vi "HTML_Build_Header_Include_Filelist.vi"(7 "rel. links (f) / include source in .html (T)":bool, 8 "Error In":errorcluster, 10 "abs Path to files on disk":path) -> (0 "Error Out":errorcluster, 1 "<head> JS":string, 2 "<head> CSS":string, 4 "JS_Scripts-Elements":string[](array[string]), 6 "CSS_Links-Elements":string[](array[string]))   [LabVIEW 2014]
uses:
  controls/HTML_Tag_Type.ctl
  controls/StylingFrameworks_Enum.ctl
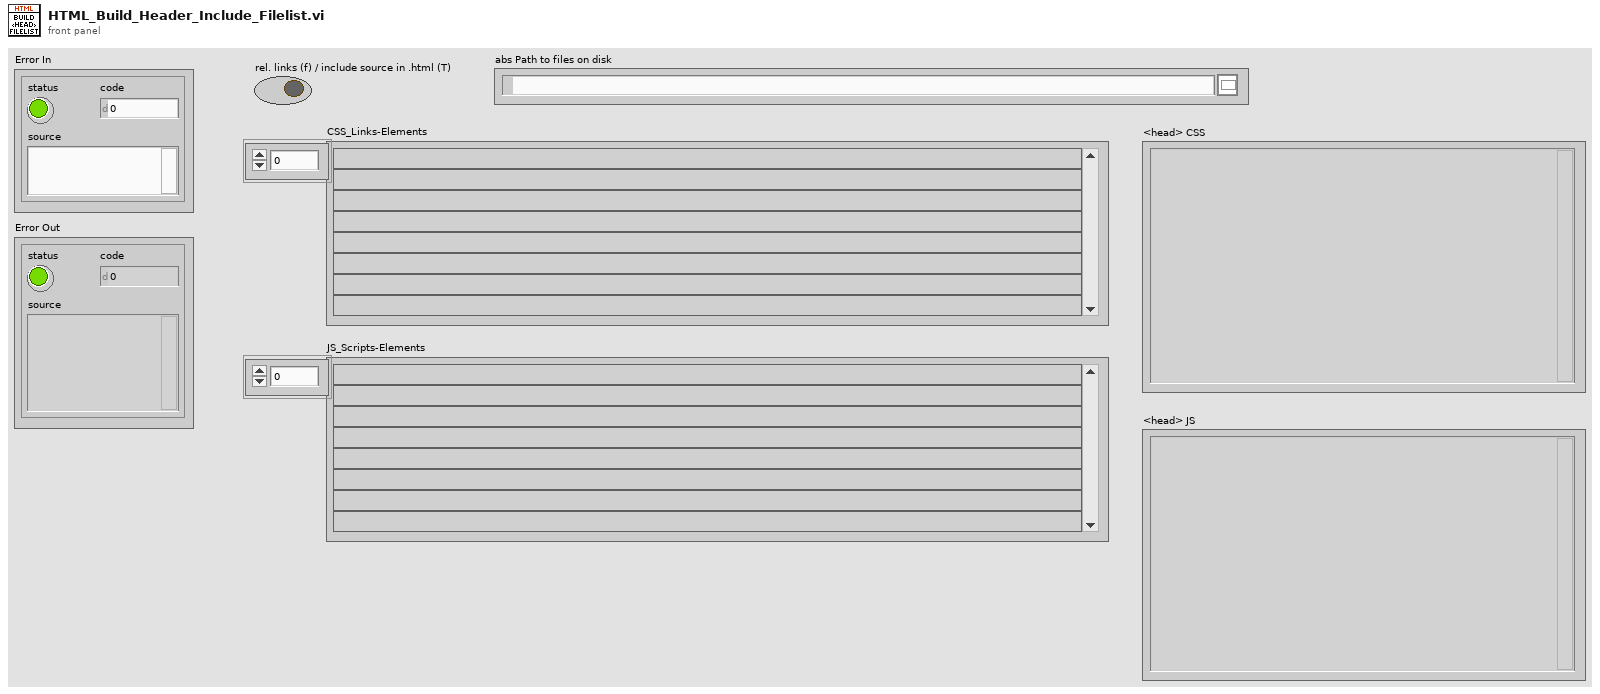
[diagram p1: front panel]
types:
  T1 = typedef "StylingFrameworks_Enum.ctl" = enum16{"None", "Bootstrap4", "Semantic-UI", "Custom"}
  T2 = typedef "HTML_Tag_Type.ctl" = enum16{"CSS-Tag", "JS-Tag"}
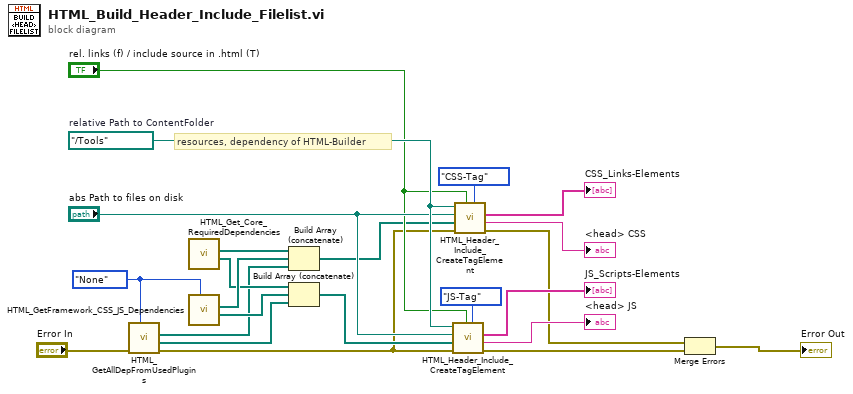
[diagram p0: block diagram]
diagram:
  w3 = StylingFrameworks_Enum."None" ("Framwork Type")
  w21 = path "../Tools"  # relative Path to ContentFolder
  # "resources, dependency of HTML-Builder"
  n1 = call "HTML_GetAllDepFromUsedPlugins.vi"("Framwork Type"=w3, "Error In"="Error In") -> ("Error Out"=w4:errorcluster, "rel. Filepaths .js"=w1:path[], "rel. Filepaths .css"=w2:path[])  [unwired: 7 in]
  n2 = call "HTML_Get_Core_RequiredDependencies.vi"() -> ("HTML_JS_General_Required_Dependencies"=w7:path[], "HTML_CSS_General_Required_Dependencies"=w11:path[])  [unwired: 10 in]
  n3 = call "HTML_GetFramework_CSS_JS_Dependencies.vi"("Framwork Type"=w3) -> ("rel. Filepaths .js"=w6:path[], "rel. Filepaths .css"=w8:path[])  [unwired: 9 in]
  n4 = Build Array (concatenate)(w11, w8, w2) -> (w10:path[])
  n5 = Build Array (concatenate)(w7, w6, w1) -> (w9:path[])
  n6 = call "HTML_Header_Include_CreateTagElement.vi"("HTML-Tag-Type"=HTML_Tag_Type."JS-Tag", "rel links (f) / include in .html (T)"="rel. links (f) / include source in .html (T)", "Error In"=w4, "rel. Filepaths .css"=w9, "abs Path to files on disk"="abs Path to files on disk", "relative Path to ContentFolder"=w21) -> ("Error Out"=w14:errorcluster, "<head> String (Out)"=→"<head> JS":string, "<head> tags[] (Out)"=→"JS_Scripts-Elements":string[])  [unwired: 3 in]
  n7 = call "HTML_Header_Include_CreateTagElement.vi"("HTML-Tag-Type"=HTML_Tag_Type."CSS-Tag", "rel links (f) / include in .html (T)"="rel. links (f) / include source in .html (T)", "Error In"=w4, "rel. Filepaths .css"=w10, "abs Path to files on disk"="abs Path to files on disk", "relative Path to ContentFolder"=w21) -> ("Error Out"=w15:errorcluster, "<head> String (Out)"=→"<head> CSS":string, "<head> tags[] (Out)"=→"CSS_Links-Elements":string[])  [unwired: 3 in]
  n8 = Merge Errors(w15, w14) -> (→"Error Out":errorcluster)
